vi "Create DCPower session.vi"(8 "error in":errorcluster, 10 "pin or relay names":string[](array[string]), 11 "Measurement Context In":refnum<class "MeasurementContext.lvclass">) -> (0 "error out":errorcluster, 1 "sessions":T2[](array[typedef]), 2 "instrument handle out":refnum<k15>, 3 "Measurement Context Out":refnum<class "MeasurementContext.lvclass">, 4 "Session manager service gRPC ID":T1, 5 "Discovery service gRPC ID":T1)   [LabVIEW 2020, in "NIDCPowerSourceDCVoltage.lvlib"]
uses:
  NIDCPowerSourceDCVoltage.lvlib
  <vilib>/MeasurementLink/MeasurementLink Measurement Server/Classes/MeasurementContext/MeasurementContext.lvclass
  <vilib>/MeasurementLink/MeasurementLink Session Management Client/RPC Messages/ni_measurementlink_sessionmanagement_v1_SessionInformation.ctl
  <vilib>/MeasurementLink/MeasurementLink Session Management Client/RPC Messages/nidevice_grpc_Session.ctl
  <vilib>/MeasurementLink/MeasurementLink Session Management Client/RPC Messages/ni_measurementlink_sessionmanagement_v1_ChannelMapping.ctl
  <vilib>/gRPC/LabVIEW gRPC Library/Shared/grpcId.ctl
  <vilib>/MeasurementLink/MeasurementLink Discovery Client/RPC Messages/ni_measurementlink_discovery_v1_ResolveServiceRequest.ctl
  <vilib>/MeasurementLink/MeasurementLink Session Management Client/RPC Messages/ni_measurementlink_sessionmanagement_v1_ReserveSessionsRequest.ctl
  <vilib>/MeasurementLink/MeasurementLink Session Management Client/RPC Messages/ni_measurementlink_PinMapContext.ctl
  <vilib>/MeasurementLink/MeasurementLink Measurement Server/MeasurementLink Measurement Server.lvlib
  <vilib>/MeasurementLink/MeasurementLink Discovery Client/MeasurementLink Discovery Client.lvlib
  <vilib>/MeasurementLink/MeasurementLink Session Management Client/MeasurementLink Session Management Client.lvlib
  <vilib>/gRPC/LabVIEW gRPC Library/grpc-lvsupport-release.lvlib
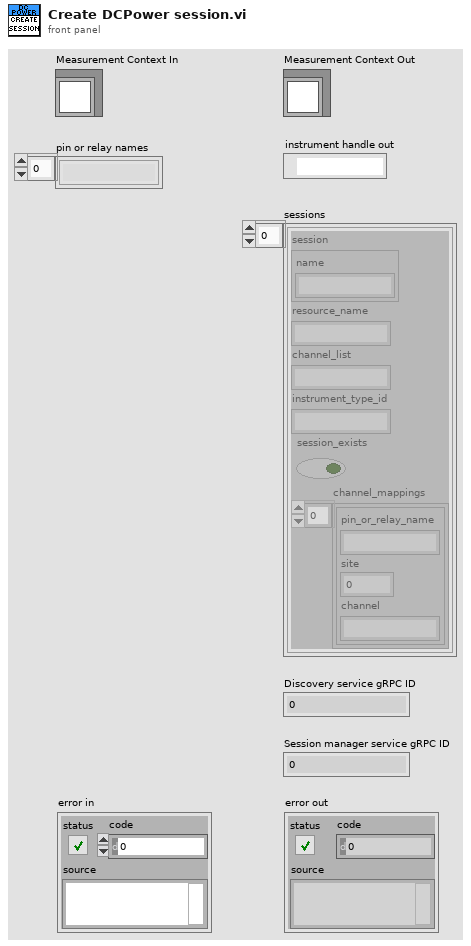
[diagram p1: front panel]
types:
  T1 = typedef "grpc-lvsupport-release.lvlib/grpcId.ctl" = u64
  T2 = typedef "MeasurementLink Session Management Client.lvlib/ni_measurementlink_sessionmanagement_v1_SessionInformation.ctl" = cluster{"session":T3, "resource_name":string, "channel_list":string, "instrument_type_id":string, "session_exists":bool, "channel_mappings":T4[]}
  T3 = typedef "MeasurementLink Session Management Client.lvlib/nidevice_grpc_Session.ctl" = cluster{"name":string}
  T4 = typedef "MeasurementLink Session Management Client.lvlib/ni_measurementlink_sessionmanagement_v1_ChannelMapping.ctl" = cluster{"pin_or_relay_name":string, "site":i32, "channel":string}
  T5 = typedef "MeasurementLink Session Management Client.lvlib/ni_measurementlink_sessionmanagement_v1_ReserveSessionsRequest.ctl" = cluster{"pin_map_context":T6, "pin_or_relay_names":string[], "instrument_type_id":string, "timeout_in_milliseconds":i32}
  T6 = typedef "MeasurementLink Session Management Client.lvlib/ni_measurementlink_PinMapContext.ctl" = cluster{"pin_map_id":string, "sites":i32[]}
  T7 = typedef "MeasurementLink Discovery Client.lvlib/ni_measurementlink_discovery_v1_ResolveServiceRequest.ctl" = cluster{"provided_interface":string, "service_class":string}
  T8 = typedef "MeasurementLink Measurement Server Internal.lvlib/ni_measurementlink_PinMapContext.ctl" = cluster{"pin_map_id":string, "sites":i32[]}
  T9 = typedef "MeasurementLink Discovery Client.lvlib/ni_measurementlink_discovery_v1_ServiceLocation.ctl" = cluster{"location":string, "insecure_port":string, "ssl_authenticated_port":string}
  T10 = typedef "MeasurementLink Session Management Client.lvlib/ni_measurementlink_sessionmanagement_v1_ReserveSessionsResponse.ctl" = cluster{"sessions":T2[]}
  T11 = typedef "niDCPower gRPC Device Server.ctl" = cluster{"session name":string, "address (localhost)":string, "port (31763)":u32}
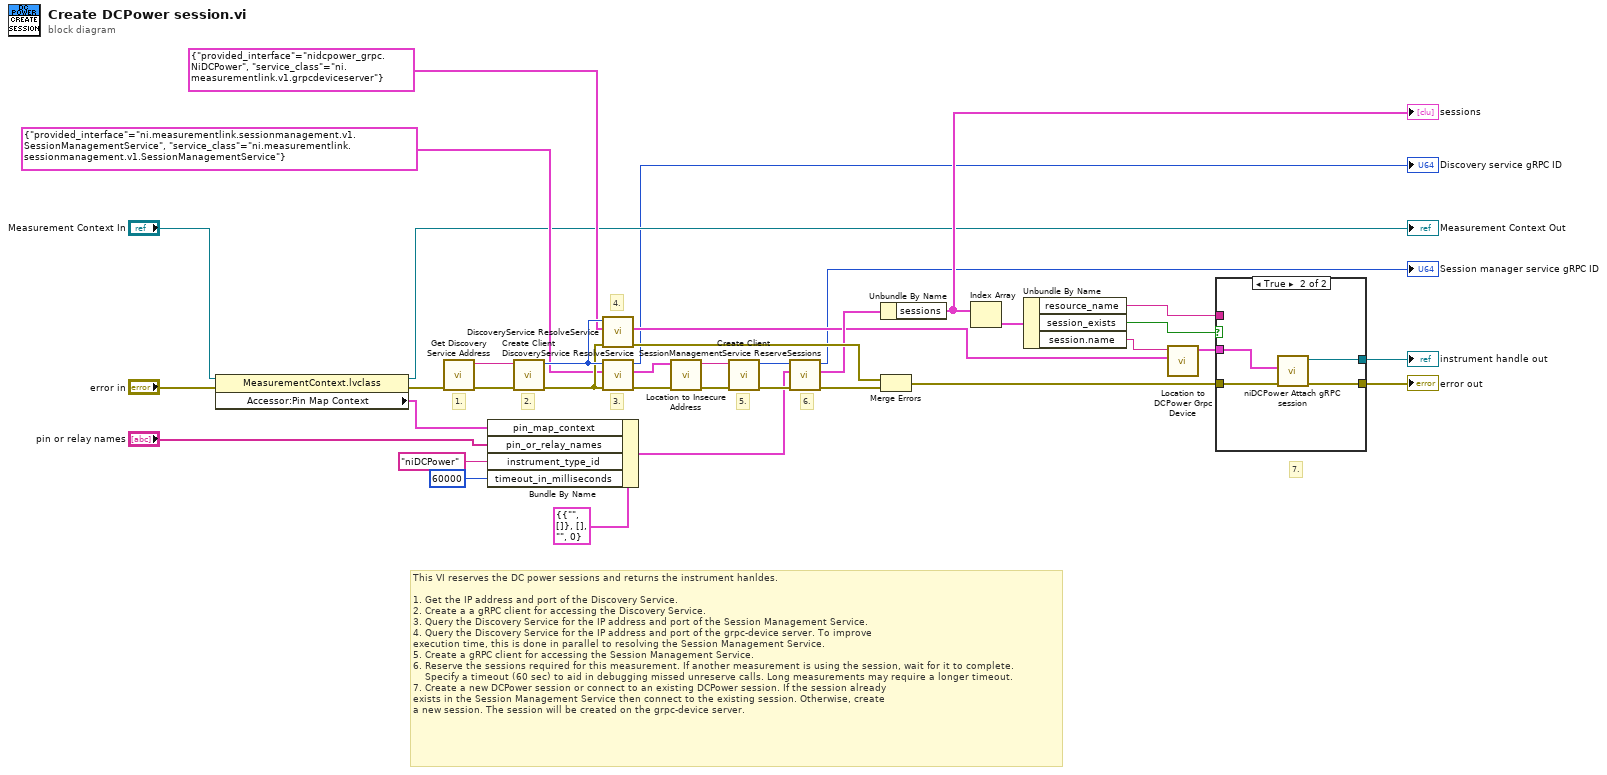
[diagram p0: block diagram]
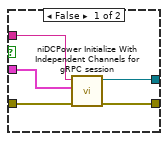
[diagram p2: hidden frame]
diagram:
  # "7."
  # "6."
  # "5."
  # "4."
  # "3."
  # "2."
  # "1."
  # "This VI reserves the DC power sessions and returns the instrument hanldes.\n\n1. Get the IP address and port of the Discovery Service.\n2. Create a a gRPC client for accessing the Discovery Service.\n3. Query the Discovery Service for the IP address and port of the Session Management Service.\n4. Query the Discovery Service for the IP address and port of the grpc-device server. To improve \nexecution time, this is done in parallel to resolving the Session Management Service.\n5. Create a gRPC client for accessing the Session Management Service.\n6. Reserve the sessions required for this measurement. If another measurement is using the session, wait for it to complete. \n    Specify a timeout (60 sec) to aid in debugging missed unreserve calls. Long measurements may require a longer timeout.\n7. Create a new DCPower session or connect to an existing DCPower session. If the session already\nexists in the Session Management Service then connect to the existing session. Otherwise, create\na new session. The session will be created on the grpc-device server."
  n1 = property class="MeasurementContext.lvclass"(reference="Measurement Context In", error in="error in") -> (reference out=→"Measurement Context Out":refnum<class "MeasurementContext.lvclass">, error out=w9:errorcluster, "Accessor:Pin Map Context"=w6:T8)
  n2 = call <vilib>:"Get Discovery Service Address.vi"("error in"=w9) -> ("error out"=w36:errorcluster, "address"=w35:string)  [unwired: 9 in]
  n3 = Bundle By Name(cluster=T5 {"pin_map_context"={"pin_map_id"="", "sites"=[]}, "pin_or_relay_names"=[], "instrument_type_id"="", "timeout_in_milliseconds"=0} ("Request Data"), "pin_map_context"=w6, "pin_or_relay_names"="pin or relay names", "instrument_type_id"="niDCPower" ("Instrument Type Id"), "timeout_in_milliseconds"=60000) -> (w5:T5)
  n4 = call <vilib>:"Create Client.vi"("error in"=w36, "address"=w35) -> ("error out"=w26:errorcluster, "gRPC ID Out"=w27:T1)  [unwired: 8 in]
  n5 = call <vilib>:"DiscoveryService ResolveService.vi"("error in"=w26, "Request Data"=T7 {"provided_interface"="nidcpower_grpc.NiDCPower", "service_class"="ni.measurementlink.v1.grpcdeviceserver"}, "gRPC ID"=w27) -> ("error out"=w29:errorcluster, "Response Data"=w4:T9)  [unwired: 6 in, 1 out]
  n6 = call <vilib>:"DiscoveryService ResolveService.vi"("error in"=w26, "Request Data"=T7 {"provided_interface"="ni.measurementlink.sessionmanagement.v1.SessionManagementService", "service_class"="ni.measurementlink.sessionmanagement.v1.SessionManagementService"}, "gRPC ID"=w27) -> ("error out"=w30:errorcluster, "Response Data"=w34:T9, "gRPC ID out"=→"Discovery service gRPC ID":T1)  [unwired: 6 in]
  n7 = call "Location to Insecure Address.vi"("Response Data"=w34) -> ("String"=w33:string)  [unwired: 10 in]
  n8 = call <vilib>:"Create Client.vi"("error in"=w30, "address"=w33) -> ("error out"=w31:errorcluster, "gRPC ID Out"=w32:T1)  [unwired: 8 in]
  n9 = call <vilib>:"SessionManagementService ReserveSessions.vi"("error in"=w31, "Request Data"=w5, "gRPC ID"=w32) -> ("error out"=w28:errorcluster, "Response Data"=w18:T10, "gRPC ID out"=→"Session manager service gRPC ID":T1)  [unwired: 6 in]
  n10 = Unbundle By Name(w18) -> ("sessions"=w17:T2[])
  "sessions" <- w17
  n11 = Merge Errors(w29, w28) -> (w16:errorcluster)
  n12 = Index Array(array=w17) -> (element=w20:T2)  [unwired: 1 in]
  n13 = Unbundle By Name(w20) -> ("resource_name"=w22:string, "session_exists"=w19:bool, "session.name"=w21:string)
  n14 = call "Location to DCPower Grpc Device.vi"("Grpc Device Location"=w4, "Session Name"=w21) -> ("NI gRPC Device Server Out"=w23:T11)  [unwired: 9 in]
  n15 = case shown="True" w19 {
    tunnel: w23 -> [w41 w45]
    tunnel: w22 -> [w40 _]
    tunnel: w16 -> [w39 w44]
    tunnel: [w38 w43] -> w15
    tunnel: [w37 w42] -> w14
    frame False {
      n16 = call <instrlib>:"niDCPower Initialize With Independent Channels for gRPC session.vi"("error in (no error)"=w39, "gRPC options"=w41, "resource name"=w40) -> ("error out"=w38:errorcluster, "instrument handle out"=w37:refnum<k15>)  [unwired: 7 in]
    }
    frame True {
      n17 = call <instrlib>:"niDCPower Attach gRPC session.vi"("error in (no error)"=w44, "gRPC options"=w45) -> ("error out"=w43:errorcluster, "instrument handle out"=w42:refnum<k15>)  [unwired: 8 in]
    }
  }
  "error out" <- w15
  "instrument handle out" <- w14
